vi "Tosca-Setup Masker.vi"(0 "Masker in":refnum<class "Channel.lvclass">, 2 "Parent VI":refnum<vi>, 5 "Use masker in":bool, 9 "Fs (Hz)":dbl) -> (4 "Masker out":refnum<class "Channel.lvclass">, 6 "Use masker out":bool, 8 "Canceled?":bool)   [LabVIEW 2020]
uses:
  epl-vi-lib/Signal Synthesis VIs/4th Generation/Controls/Channel/Channel.xctl
  epl-vi-lib/Signal Synthesis VIs/4th Generation/Classes/Channel/Channel.lvclass
  epl-vi-lib/Utility VIs/Buttons/KCheckmarkBoolean 2.ctl
  Sub VIs/Tosca-Globals.vi
panel:
  in  "Use masker":T1
  in  "Channel":refnum<class "Channel.lvclass">(xcontrol)
  in  "Message":string="Note: masker channel must be the only input or output on its DAQ board."
  in  "Cancel":bool
  in  "OK":bool
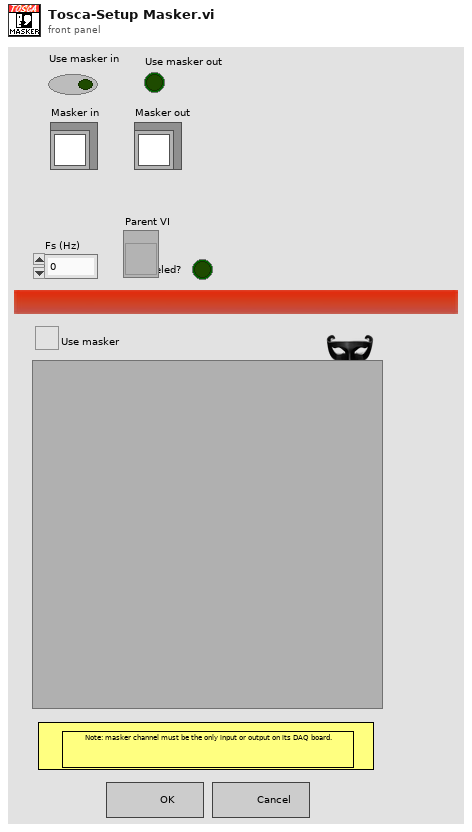
[diagram p1: front panel]
types:
  T1 = typedef "KCheckmarkBoolean 2.ctl" = bool
  T2 = enum8{"Enabled", "Disabled", "Disabled and Grayed Out"}
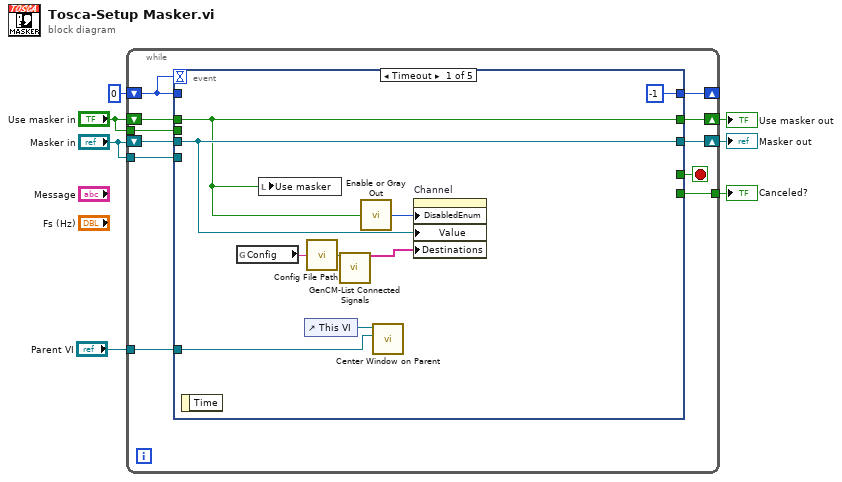
[diagram p0: block diagram]
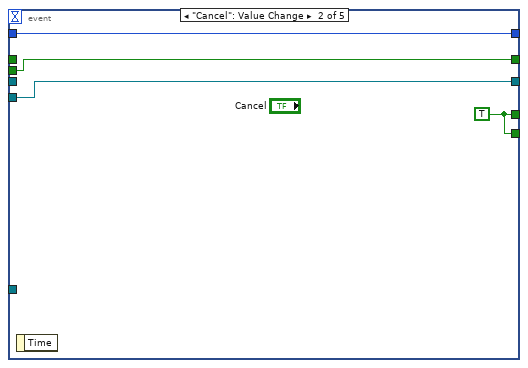
[diagram p2: hidden frame]
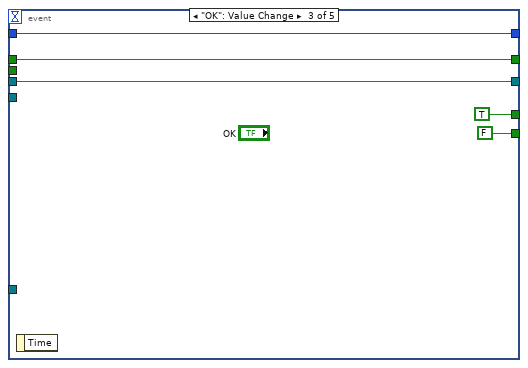
[diagram p3: hidden frame]
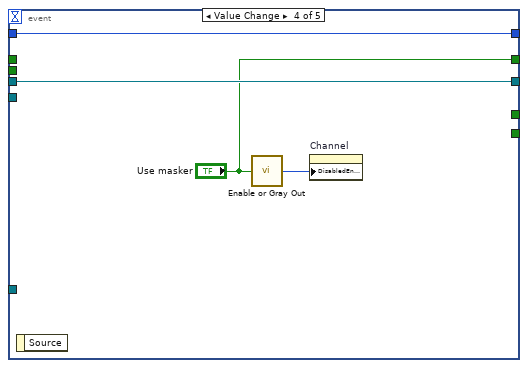
[diagram p4: hidden frame]
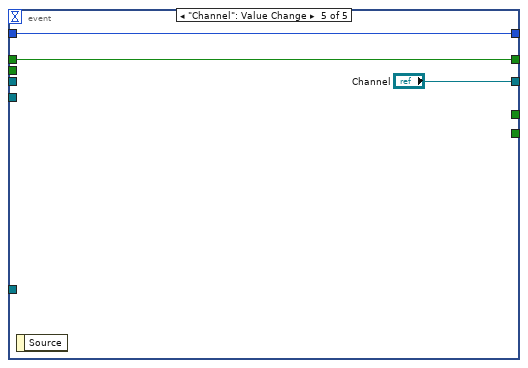
[diagram p5: hidden frame]
diagram:
  n1 = while {
    shift-right: [w18] -> _
    shift-left: 0 -> [w11]
    tunnel: [w15] -> w6
    shift-right: [w12] -> w5
    shift-left: "Masker in" -> [w13]
    shift-right: [w17] -> w4
    shift-left: "Use masker in" -> [w14]
    tunnel: "Use masker in" -> [w10]
    tunnel: "Masker in" -> [w9]
    tunnel: "Parent VI" -> [w8]
    stop <- w16 stop-if-true
    n2 = event shown="[0] Timeout" {
      selector: _ -> [_ _ _ _ _]
      dyn-events: _ -> [_ _ _ _ _]
      timeout: w11 -> [_ _ _ _ _]
      tunnel: [-1 w28 w34 w39 w43] -> w18
      tunnel: w14 -> [w25 _ w33 _ w42]
      tunnel: [w25 w30 w33 "Use masker" w42] -> w17
      tunnel: [_ w31 TRUE _ _] -> w16
      tunnel: [_ w31 FALSE _ _] -> w15
      tunnel: w13 -> [w26 _ w32 w40 _]
      tunnel: [w26 w29 w32 w40 "Channel"] -> w12
      tunnel: w11 -> [_ w28 w34 w39 w43]
      tunnel: w10 -> [_ w30 _ _ _]
      tunnel: w9 -> [_ w29 _ _ _]
      tunnel: w8 -> [w22 _ _ _ _]
      event Timeout {
        n3 = event-data() -> ()  [unwired: 1 in, 1 out]
        n4 = global read "Tosca-Globals.vi" "Config"() -> (w21:string)
        n5 = local write "Use masker"(w25) -> ()
        n6 = control-ref of="This VI"() -> (w23:refnum<vi>)
        n7 = call "Config File Path.vi"("AppName"=w21) -> ("Default config file name"=w20:path)
        n8 = call "GenCM-List Connected Signals.vi"("Path"=w20) -> ("Analog Outputs"=w19:string[])  [unwired: 10 in, 4 out]
        n9 = call "Enable or Gray Out.vi"("Boolean"=w25) -> ("Disabled"=w24:T2)
        n10 = call "Center Window on Parent.vi"("Parent VI"=w22, "VI in"=w23) -> ()  [unwired: 8 in, 2 out]
        n11 = property on="Channel" class="Channel (strict)"("DisabledEnum"=w24, "Value"=w26, "Destinations"=w19) -> ()  [unwired: 2 in, 2 out]
      }
      event "Cancel": Value Change {
        w31 = TRUE
        n12 = event-data() -> ()  [unwired: 1 in, 1 out]
      }
      event "OK": Value Change {
        n13 = event-data() -> ()  [unwired: 1 in, 1 out]
      }
      event Value Change {
        n14 = event-data() -> ()  [unwired: 1 in, 1 out]
        n15 = call "Enable or Gray Out.vi"("Boolean"="Use masker") -> ("Disabled"=w37:T2)
        n16 = property on="Channel" class="Channel (strict)"("DisabledEnum"=w37) -> ()  [unwired: 2 in, 2 out]
      }
      event "Channel": Value Change {
        n17 = event-data() -> ()  [unwired: 1 in, 1 out]
      }
    }
  }
  "Canceled?" <- w6
  "Use masker out" <- w4
  "Masker out" <- w5
